vi "Flush Buffer Data to File.vi"(5 "Channel Names":string[](array[string]), 6 "dt":dbl, 7 "Group Names":string[](array[string]), 8 "error in (no error)":errorcluster, 9 "Waveform":bool, 10 "Buffer Data in":T1, 11 "Segmented Log Ref in":refnum<data-value>) -> (0 "error out":errorcluster, 1 "Log Completed":bool, 2 "Buffer Data out":T1, 3 "Segmented Log Ref out":refnum<data-value>)   [LabVIEW 2012, in "Triggered Log.lvclass"]
doc: "Flushes any data in the buffer to the segmented log file. This VI has no effect if the buffer is emtpy. This VI checks if the position pointer for the buffer has wrapped around when used as a circular buffer by checking if the position pointer and the length of the used portion of the buffer are not in phase. The position pointer starts over at zero after the final element, but the length saturates at the max length of the buffer. This allows us to know when the buffer has wrapped around."
uses:
  Triggered Log.lvclass
  Engine/Classes/Logs/Segmented Logs/Segmented Log/Segmented Log.lvclass
  Buffer Data.ctl
  Engine/Classes/Logs/Segmented Logs/Segmented Log/Segmented Log.lvclass/Segmented Log.ctl
  Shared/Classes/Log File Specifications/Log File Specification/Log File Specification.lvclass/Log File Specification.ctl
  Engine/Classes/Logs/Segmented Logs/Segmented Log/Check Close File.vi
  Engine/Classes/Logs/Segmented Logs/Segmented Log/Check Open File.vi
  Engine/Classes/Logs/Segmented Logs/Segmented Log/Close Log File Instance.vi
  Engine/Classes/Logs/Segmented Logs/Segmented Log/Open Log File Instance.vi
  Engine/Classes/Logs/Segmented Logs/Segmented Log/On Segmented Log Complete.vi
  Engine/Classes/Logs/Segmented Logs/Segmented Log/On File Close.vi
  Shared/Classes/Log File Specifications/Log File Specification/Open Log File.vi
  Shared/Classes/Log File Specifications/Log File Specification/Set Path Tag.vi
  Engine/Classes/Logs/Segmented Logs/Segmented Log/On File Open.vi
  Shared/Classes/Log File Specifications/Log File Specification/Set Filename Offset.vi
  Shared/Classes/Log File Specifications/Log File Specification/Build File Path.vi
  Shared/Classes/Log File Specifications/Log File Specification/Resolve File Conflicts.vi
  Shared/Classes/Log File Specifications/Log File Specification/Initialize Log File.vi
  <vilib>/Utility/libraryn.llb/Check if File or Folder Exists.vi
  <vilib>/Utility/error.llb/Error Cluster From Error Code.vi
  <vilib>/Utility/libraryn.llb/Get File Extension.vi
  <vilib>/Utility/libraryn.llb/Create Directory Recursive.vi
  Engine/Classes/Logs/Log Files/Log File/Write to Log File (Waveform).vi
  Engine/Classes/Logs/Segmented Logs/Segmented Log/Segment Log File.vi
  Engine/Classes/Logs/Log Files/Log File/Close Log File.vi
  Engine/Classes/Logs/Segmented Logs/Segmented Log/Make File Read-Only.vi
  Engine/Classes/Logs/Log Files/Log File/Write to Log File.vi
  Engine/Classes/Logs/Log Files/Log File/Log File.lvclass
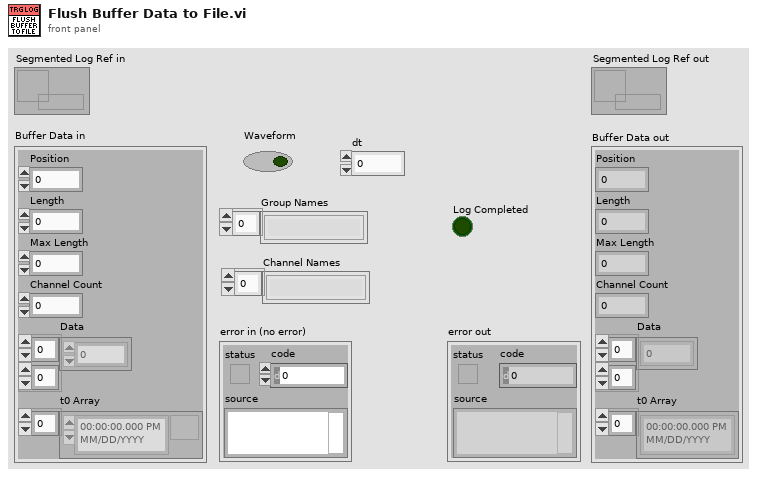
[diagram p1: front panel]
types:
  T1 = typedef "Triggered Log.lvclass/Buffer Data.ctl" = cluster{"Position":i32, "Length":i32, "Max Length":i32, "Channel Count":i32, "Data":dbl[][], "t0 Array":timestamp[]}
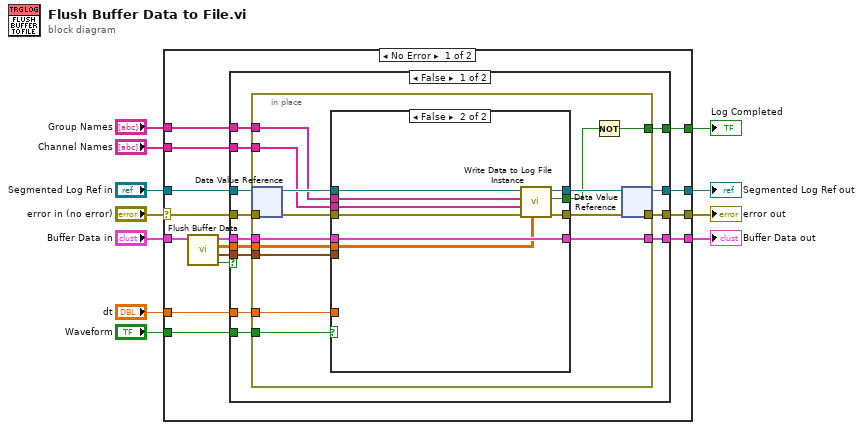
[diagram p0: block diagram]
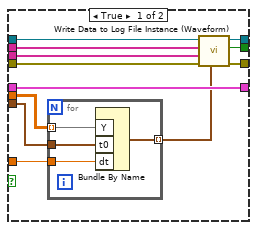
[diagram p2: hidden frame]
diagram:
  n1 = case shown="No Error" "error in (no error)" {
    selector: "error in (no error)" -> [w26 w84]
    tunnel: [w25 w84] -> w10
    tunnel: "Buffer Data in" -> [w20 w82]
    tunnel: "Segmented Log Ref in" -> [w24 w83]
    tunnel: [w23 w83] -> w8
    tunnel: "Group Names" -> [w22 _]
    tunnel: "Channel Names" -> [w21 _]
    tunnel: [w19 w82] -> w4
    tunnel: [w16 _] -> w3
    tunnel: "Waveform" -> [w14 _]
    tunnel: "dt" -> [w12 _]
    frame No Error {
      n2 = call "Flush Buffer Data.vi"("Buffer Data in"=w20) -> ("Buffer Empty"=w15:bool, "t0"=w13:timestamp, "Buffer Data"=w18:dbl[][], "Buffer Data out"=w17:T1)  [unwired: 7 in]
      n3 = case shown="False" w15 {
        tunnel: w26 -> [w39 w80]
        tunnel: [w38 w80] -> w25
        tunnel: w24 -> [w37 w81]
        tunnel: [w36 w81] -> w23
        tunnel: w22 -> [w35 _]
        tunnel: w21 -> [w34 _]
        tunnel: w18 -> [w33 _]
        tunnel: [w32 w79] -> w19
        tunnel: w17 -> [w31 w79]
        tunnel: [w30 _] -> w16
        tunnel: w14 -> [w29 _]
        tunnel: w13 -> [w28 _]
        tunnel: w12 -> [w27 _]
        frame False {
          n4 = in-place {
            in-place-border: w39 -> [_]
            in-place-border: [w51] -> w38
            in-place-border: w35 -> [w50]
            in-place-border: w34 -> [w49]
            in-place-border: w33 -> [w47]
            in-place-border: [w40] -> w32
            in-place-border: w31 -> [w41]
            in-place-border: [w45] -> w30
            in-place-border: w29 -> [w44]
            in-place-border: w28 -> [w43]
            in-place-border: w27 -> [w42]
            n5 = in-place-dvr #1(w37) -> (w52:refnum<class "Segmented Log.lvclass">, w53:errorcluster)
            n6 = case shown="False" w44 {
              tunnel: w53 -> [w64 w77]
              tunnel: w52 -> [w63 w76]
              tunnel: [w62 w75] -> w51
              tunnel: w50 -> [w61 w74]
              tunnel: w49 -> [w60 w73]
              tunnel: [w59 w72] -> w48
              tunnel: w47 -> [w57 w71]
              tunnel: [w58 w70] -> w46
              tunnel: w43 -> [w56 _]
              tunnel: w42 -> [w55 _]
              tunnel: w41 -> [w65 w78]
              tunnel: [w65 w78] -> w40
              frame True {
                n7 = for {
                  tunnel: w57 -> [w69] mode=indexing
                  tunnel: w56 -> [w68]
                  tunnel: w55 -> [w67]
                  tunnel: [w66] -> w54 mode=indexing
                  n8 = Bundle By Name("Y"=w69, "t0"=w68, "dt"=w67) -> (w66:waveform(dbl))  [unwired: 1 in]
                }
                n9 = call "Write Data to Log File Instance (Waveform).vi"("Waveform Data"=w54, "error in (no error)"=w64, "Channel Names"=w60, "Group Names"=w61, "Segmented Log in"=w63) -> ("error out"=w62:errorcluster, "Log Active"=w58:bool, "Segmented Log out"=w59:refnum<class "Segmented Log.lvclass">)  [unwired: 4 in]
              }
              frame False {
                n10 = call "Write Data to Log File Instance.vi"("Data"=w71, "error in (no error)"=w77, "Channel Names"=w73, "Group Names"=w74, "Segmented Log in"=w76) -> ("error out"=w75:errorcluster, "Log Active"=w70:bool, "Segmented Log out"=w72:refnum<class "Segmented Log.lvclass">)  [unwired: 4 in]
              }
            }
            n11 = Not(x=w46) -> (.not. x?=w45:bool)
            n12 = in-place-dvr #1(w48) -> (w36:refnum<data-value>)  [unwired: 1 out]
          }
        }
        frame True {
          # "The buffer is empty. Do nothing."
        }
      }
    }
    frame Error {
    }
  }
  "error out" <- w10
  "Segmented Log Ref out" <- w8
  "Buffer Data out" <- w4
  "Log Completed" <- w3
